vi "Mood Override.vi"(10 "Mood Override in":string, 11 "Mood Override Counter in":u32) -> (2 "Mood Override out":string, 3 "Mood Override Counter out":u32)   [LabVIEW 2026]
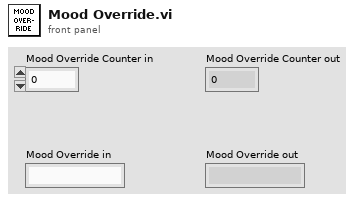
[diagram p1: front panel]
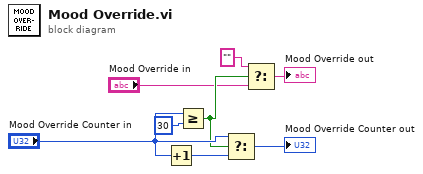
[diagram p0: block diagram]
diagram:
  n1 = Increment(x="Mood Override Counter in") -> (x+1=w6:u32)
  n2 = Greater Or Equal?(x="Mood Override Counter in", y=u32 30) -> (x >= y?=w4:bool)
  n3 = Select(t="Mood Override Counter in", s=w4, f=w6) -> (s? t:f=→"Mood Override Counter out":u32)
  n4 = Select(t="", s=w4, f="Mood Override in") -> (s? t:f=→"Mood Override out":string)
